vi "Client.vi"() -> ()   [LabVIEW 2015]
doc: "This VI implements a client for the TCP Named Service - Server.vi. It connects to a service by specifying the server address and the name of the service. The client receives the string sent by the server, displays the string and closes the connection."
panel:
  out "Message from Server":string
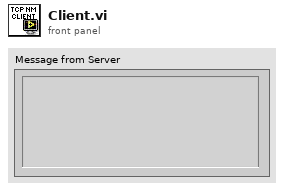
[diagram p1: front panel]
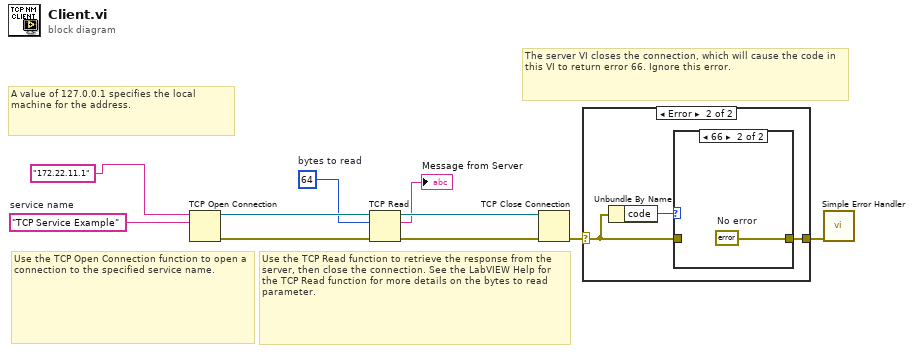
[diagram p0: block diagram]
diagram:
  w4 = 64  # bytes to read
  w5 = "TCP Service Example"  # service name
  # "The server VI closes the connection, which will cause the code in this VI to return error 66. Ignore this error."
  # "A value of 127.0.0.1 specifies the local machine for the address."
  # "Use the TCP Open Connection function to open a connection to the specified service name."
  # "Use the TCP Read function to retrieve the response from the server, then close the connection. See the LabVIEW Help for the TCP Read function for more details on the bytes to read parameter."
  n1 = TCP Open Connection(address="172.22.11.1" ("IP"), remote port or service name=w5) -> (connection ID=w9:refnum<k5>, error out=w10:errorcluster)  [unwired: 3 in]
  n2 = TCP Read(connection ID=w9, bytes to read=w4, error in (no error)=w10) -> (connection ID out=w8:refnum<k5>, data out=→"Message from Server":string, error out=w7:errorcluster)  [unwired: 2 in]
  n3 = TCP Close Connection(connection ID=w8, error in (no error)=w7) -> (error out=w3:errorcluster)  [unwired: 1 in, 1 out]
  n4 = case shown="Error" w3 {
    selector: w3 -> [w11 w13]
    tunnel: [w11 w12] -> w2
    frame No Error {
    }
    frame Error {
      n5 = Unbundle By Name(w13) -> ("code"=w14:i32)
      n6 = case shown="66" w14 {
        tunnel: w13 -> [w15 _]
        tunnel: [w15 w16] -> w12
        frame Default {
        }
        frame 66 {
          w16 = errorcluster {"status"=FALSE, "code"=0, "source"=""}  # No error
        }
      }
    }
  }
  n7 = call <vilib>:"Simple Error Handler.vi"("error in (no error)"=w2) -> ()  [unwired: 4 in, 5 out]
